vi "menuItemsWorkaround_rec.vi"() -> (1 "timed out?":bool, 3 "flatMenu[]":T1)   [LabVIEW 2013]
uses:
  flatMenu.ctl
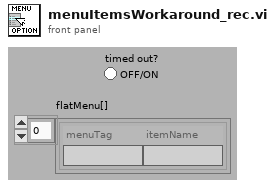
[diagram p1: front panel]
types:
  T1 = typedef "flatMenu.ctl" = cluster{"menuTag":string, "itemName":string}[]
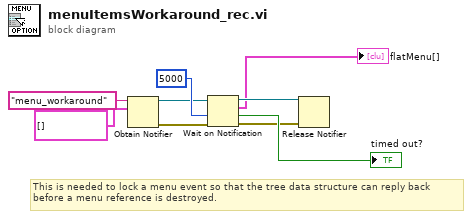
[diagram p0: block diagram]
diagram:
  # "This is needed to lock a menu event so that the tree data structure can reply back \nbefore a menu reference is destroyed."
  n1 = Obtain Notifier(name (unnamed)="menu_workaround", notification data type=T1 [] ("flatMenu[]")) -> (notifier out=w4:refnum<notifier>, error out=w5:errorcluster)  [unwired: 2 in, 1 out]
  n2 = Wait on Notification(notifier=w4, timeout in ms (-1)=5000, error in (no error)=w5) -> (notifier out=w7:refnum<notifier>, notification=→"flatMenu[]":T1, timed out?=→"timed out?":bool, error out=w8:errorcluster)  [unwired: 1 in]
  n3 = Release Notifier(notifier=w7, error in (no error)=w8) -> ()  [unwired: 1 in, 3 out]
